vi "Skyline Send Waveform File.vi"(8 "error in":errorcluster, 9 "properties":cluster{"Key":string, "Value":string}[](array[cluster]) caption="properties (null)", 11 "data in":waveform(dbl)[](array[waveform])) -> (0 "error out":errorcluster, 2 "size in bytes":i32, 3 "data out":waveform(dbl)[](array[waveform]))   [LabVIEW 2016]
uses:
  <vilib>/FileIngestion/Close (Single).vi
  <vilib>/FileIngestion/FileIngestion.lvlib
  <resource>/objmgr/FileIngestion.rc
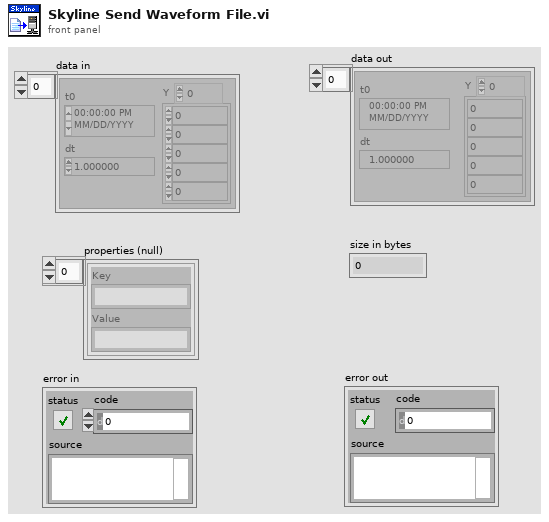
[diagram p1: front panel]
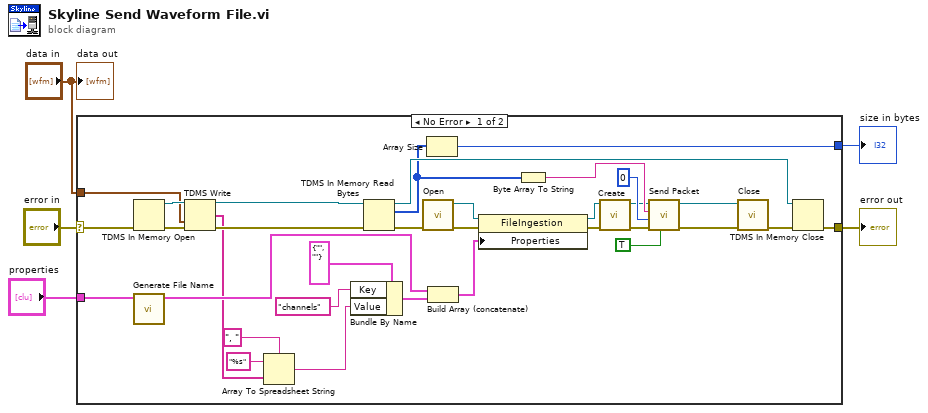
[diagram p0: block diagram]
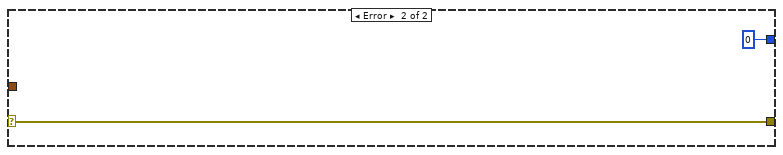
[diagram p2: hidden frame]
diagram:
  n1 = case shown="No Error" "error in" {
    selector: "error in" -> [w26 w40]
    tunnel: [w28 w40] -> w5
    tunnel: "properties" -> [w38 _]
    tunnel: "data in" -> [w36 _]
    tunnel: [w24 0] -> w1
    frame No Error {
      n2 = TDMS In Memory Open(8:w26) -> (0:w27:errorcluster, 3:w37:refnum<k34>)  [unwired: 1 in]
      n3 = call "Generate File Name.vi"("properties"=w38) -> ("Array"=w13:cluster{"Key":string, "Value":string}[])  [unwired: 10 in]
      n4 = TDMS Write(0:w37, 9:w36, 11:w27) -> (4:w15:refnum<k34>, 8:w10:string[], 15:w35:errorcluster)  [unwired: 3 in, 1 out]
      n5 = Array To Spreadsheet String(delimiter (Tab)=", ", array=w10, 3:"%s" ("format string")) -> (spreadsheet string=w6:string)
      n6 = Bundle By Name(cluster=cluster{"Key":string, "Value":string} {"Key"="", "Value"=""} ("Property"), "Key"="channels", "Value"=w6) -> (w12:cluster{"Key":string, "Value":string})
      n7 = TDMS In Memory Read Bytes(8:w35, 11:w15) -> (0:w32:errorcluster, 2:w25:u8[], 3:w34:refnum<k34>)  [unwired: 2 in]
      n8 = call <vilib>:"Open.vi"("error in (no error)"=w32) -> ("error out"=w20:errorcluster, "file refnum"=w21:refnum<k21>)  [unwired: 9 in]
      n9 = Array Size(array=w25) -> (size(s)=w24:i32)
      n10 = Build Array (concatenate)(w13, w12) -> (w11:cluster{"Key":string, "Value":string}[])
      n11 = property class="FileIngestion"(reference=w21, error in=w20, "Properties"=w11) -> (reference out=w19:refnum<k21>, error out=w18:errorcluster)
      n12 = Byte Array To String(unsigned byte array=w25) -> (string=w33:string)
      n13 = call <vilib>:"Create.vi"("error in (no error)"=w18, "file refnum in"=w19) -> ("error out"=w17:errorcluster, "file refnum out"=w16:refnum<k21>)  [unwired: 7 in]
      n14 = call <vilib>:"Send Packet.vi"("is last packet"=TRUE, "error in (no error)"=w17, "packet number (0)"=0 ("packet number"), "data"=w33, "file refnum in"=w16) -> ("error out"=w30:errorcluster, "file refnum out"=w31:refnum<k21>)  [unwired: 5 in]
      n15 = call-poly <vilib>:"Close.vi"("error in (no error)"=w30, "file refnum in"=w31) -> ("error out"=w29:errorcluster)  [unwired: 9 in]
      n16 = TDMS In Memory Close(8:w29, 11:w34) -> (0:w28:errorcluster)  [unwired: 2 in]
    }
    frame Error {
    }
  }
  "error out" <- w5
  "size in bytes" <- w1
  "data out" <- "data in"
